vi "Igor_LoadWaveFromFile.vi"(7 "Path":path, 8 "error in (no error)":errorcluster, 9 "Wave":dbl[](array[numeric]), 10 "Wavename":string, 11 "Application":refnum<k7>) -> (0 "error out":errorcluster, 3 "Application":refnum<k7>)   [LabVIEW 2019]
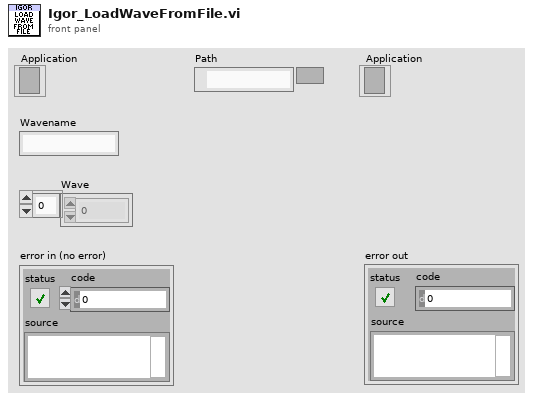
[diagram p1: front panel]
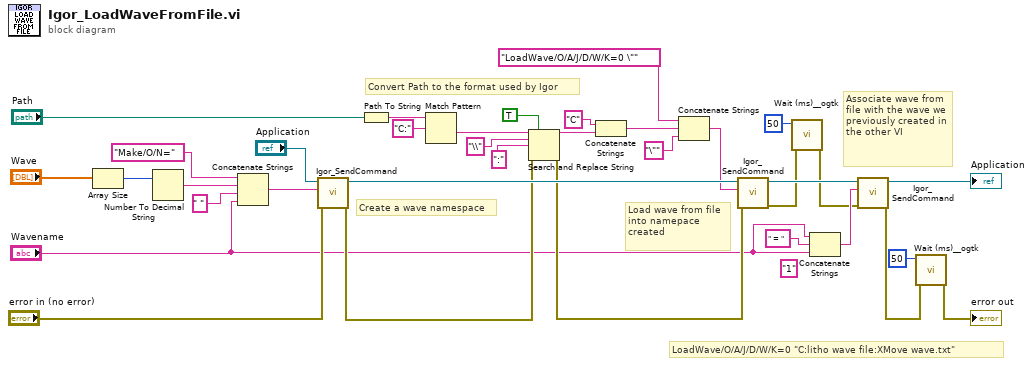
[diagram p0: block diagram]
diagram:
  (unwired) "1" ("string")
  # "Associate wave from file with the wave we previously created in the other VI"
  # "Load wave from file into namepace created"
  # "Create a wave namespace"
  # "Convert Path to the format used by Igor"
  # "LoadWave/O/A/J/D/W/K=0 \"C:litho wave file:XMove wave.txt\""
  n1 = Array Size(array="Wave") -> (size(s)=w23:i32)
  n2 = Number To Decimal String(number=w23) -> (decimal integer string=w21:string)  [unwired: 1 in]
  n3 = Concatenate Strings("Make/O/N=", w21, " " ("string"), "Wavename") -> (w25:string)
  n4 = call "Igor_SendCommand.vi"("error in (no error)"="error in (no error)", "command"=w25, "Application In"="Application") -> ("error out"=w10:errorcluster, "Application Out"=w31:refnum<k7>)  [unwired: 5 in, 2 out]
  n5 = Path To String(path="Path") -> (string=w14:string)
  n6 = Match Pattern(string=w14, regular expression="C:") -> (after substring=w18:string)  [unwired: 1 in, 3 out]
  n7 = Search and Replace String(replace all?=TRUE ("replace all? (F)"), input string=w18, search string="\\", replace string=":" ("replace string (\"\")"), error in=w10) -> (result string=w16:string, error out=w9:errorcluster)  [unwired: 3 in, 2 out]
  n8 = Concatenate Strings("C" ("string"), w16) -> (w28:string)
  n9 = Concatenate Strings("LoadWave/O/A/J/D/W/K=0 \"" ("string"), w28, "\"" ("string")) -> (w30:string)
  n10 = call "Igor_SendCommand.vi"("error in (no error)"=w9, "command"=w30, "Application In"=w31) -> ("error out"=w6:errorcluster, "Application Out"=w34:refnum<k7>)  [unwired: 5 in, 2 out]
  n11 = call <userlib>:"Wait (ms)__ogtk.vi"("error in (no error)"=w6, "milliseconds to wait"=u32 50) -> ("error out"=w5:errorcluster)  [unwired: 8 in, 1 out]
  n12 = Concatenate Strings("Wavename", " = " ("string"), "Wavename") -> (w33:string)
  n13 = call "Igor_SendCommand.vi"("error in (no error)"=w5, "command"=w33, "Application In"=w34) -> ("error out"=w3:errorcluster, "Application Out"=→"Application":refnum<k7>)  [unwired: 5 in, 2 out]
  n14 = call <userlib>:"Wait (ms)__ogtk.vi"("error in (no error)"=w3, "milliseconds to wait"=u32 50) -> ("error out"=→"error out":errorcluster)  [unwired: 8 in, 1 out]
